vi "SCMP - Data Acquisition - v6.vi"(0 "Max FPS limit":dbl=10.0 format="%.1g", 1 "LCVR Voltages":dbl[][](array[numeric]), 2 "Mod/Seq":bool, 5 "Cycles":i32=1 min=1 max=30 step=1, 7 "Save to FITS?":bool=TRUE, 9 "Headers In":T12[](array[typedef])=[{"Wavelength (nm)"=530.15, "Exposure (s)"=0.05, "Tuning Delay (ms)"=1000.0, "Beam Type (-1/1)"=1.0, "Tuning Voltages"=[1.111, 2.222, 3.333, 4.444], "Observer"="observer", "Light Shapping Diffuser"=enum."In Beam", "Comment"="", "Data Type"=9, "Mod Cycles"=0, "SCD Calibration Optics"=enum."1 - Polarizer @0, I+Q", "SCD Emission Line Filter"=enum."1-557.6nm", "Cookbook"="", "COMP-S Calibration Wheel"=enum."Dark", "COMP-S Andover Filter Wheel"=enum."530.3nm/HWB 0.34nm (Fe XIV)", "FOV Rotation (deg)"=66.0, "Objective Lens Position (mm)"=0.0, "Occulter size"=0.0, "Time End"=timestamp(3382374145.421875 s since 1904-01-01), "Acc Exposure (s)"=0.0, "Time Stamp Array"=[], "Camera Serial Number"=[], "Camera Temp"=[], "Camera PI (mm)"=[], "Time Start"=timestamp(3382374145.421875 s since 1904-01-01), "Peripherals"={"ILX controler"=FALSE, "Zone temperatures"=FALSE, "Andor"=FALSE, "Andor 2"=FALSE, "PI Stages"=FALSE, "AISAS mechanisms"=FALSE, "AISAS Mech.lvclass"=refnum, "Zone temp ref"=variant, "FWs"=FALSE}, "FITS paths"=[], "Cameras"=enum."Andor", "load preset cbk"=FALSE, "periodic check count"=0, "COMP-S Calibration Wheel 2"=enum."Dark", "Calib"=enum."Dark", "Abso Aperture"=40.0, "Nominal Aperture"=196.0}] {"Nominal Aperture" format="%.1f"; "Abso Aperture" format="%.1f"; "Camera PI (mm)" format="%_3g"; "Acc Exposure (s)" format="%^.3g"; "Occulter size" format="%.2f"; "Objective Lens Position (mm)" min=70.0 max=152.0 format="%.2f"; "FOV Rotation (deg)" format="%.1f"; "Data Type" items=["LIVE", "DARK", "FLAT", "CALI", "OBSE", "ABSO", "AURE", "TARG", "OBJE", "HOLE", "OREX", "THRO", "CHIP"]; "Exposure (s)" format="%^.3g"; "Wavelength (nm)" format="%_6g"}, 11 "error in":errorcluster, 12 "Andor Neo":T13[](array[typedef]) {"Exposure (s)" format="%^.3g"; "Time at Synch" format="%<%H:%M:%S>T"; "Interframe Time" format="%#_3g"; "Frame Readout Time" format="%_3g"; "Row Readout Time" format="%_3g"}) -> (3 "FITS Path Out":path, 6 "Image":u32[][](array[numeric]), 8 "Image 2":u32[][](array[numeric]), 10 "Headers Out":T2[](array[typedef]) {"Nominal Aperture" format="%.1f"; "Abso Aperture" format="%.1f"; "Camera PI (mm)" format="%_3g"; "Acc Exposure (s)" format="%^.3g"; "Occulter size" format="%.2f"; "Objective Lens Position (mm)" min=70.0 max=152.0 format="%.2f"; "FOV Rotation (deg)" format="%.1f"; "Exposure (s)" format="%^.3g"; "Wavelength (nm)" format="%_6g"}, 13 "FITS Path Out 2":path, 15 "error out":errorcluster)   [LabVIEW 2014]
doc: "The LL Sequence VI acquires a sequence of images and displays them in an array of image controls using the low-level acquisition VIs. A sequence is appropriate for applications that process multiple images. You can configure a sequence to acquire every frame or to skip a variable number of frames between each image.\n\nTop Level Code Overview\n1) Initialize Camera (Global Shutter, High Well, Low Noise, exposure time, etc.)\n2) Create a buffer set equal in size to the # of trigger pulses (e.g. 100) which is the same as the # of expected images \n3) Start the camera acquisition THEN start the DAQmx task (use merge error cluster to gurantee this)"
uses:
  Controls/run cbk timeout.ctl
  Controls/Globals.vi
  <vilib>/Waveform/WDTOps.llb/WDT Waveform Duration DBL.vi
  <vilib>/DAQmx/write.llb/DAQmx Write (Analog 1D Wfm NChan NSamp).vi
  <vilib>/DAQmx/create/channels.llb/DAQmx Create Channel (AO-Voltage-Basic).vi
  <vilib>/DAQmx/configure/timing.llb/DAQmx Timing (Use Waveform).vi
  Controls/SCD - Calibration Optics Filter Wheel.ctl
  AISAS/Controls/Diffuser.ctl
  Controls/SCD - FITS Cluster.ctl
  Camera/Andor Neo Info.ctl
  Controls/SCD - EDT - Emission Line Filter Wheel.ctl
  Controls/CoMP-S Controls/Polarization Optics Filter Wheel.ctl
  Controls/CoMP-S Controls/Emission Line Filter Wheel.ctl
  AISAS/Controls/focus.ctl
  Controls/beaning.ctl
  AISAS/Mech/AISAS Mech.lvclass
  Controls/peripherals.ctl
  Controls/Cameras select.ctl
  Controls/FITS Data type.ctl
panel:
  out "error Andor queue":errorcluster
  out "error cam dequeue & queue RAM 2":errorcluster
  out "error dequeue RAM 2":errorcluster
  out "seq cycles":i32=1
  out "error proc queue":errorcluster
  out "mod cycles *4":i32=1
  out "error RAM queue":errorcluster
  in  "count 2":i32
  in  "Tab Control":T1(tab)
  out "FPS":dbl=10.0 format="%.1g"
  out "Camera T Image":u32[][](graph)
  out "# Images in queue":i32
  out "Image Acq (s)":dbl(slide)=4151.832132564842
  out "Image Processing":i32(slide) scale=-1.0..11.0
  in  "user break":bool
  out "Camera R Image":u32[][](graph)
  out "Camera T Image Zoom":u32[][](graph)
  out "# Images to acquire":i32
  out "Image Acq Started":bool
  in  "image pointers":u64[](array[numeric])
  in  "imageNo":i32 caption="Image No"
  in  "count":i32
  out "# Wavelengths":i32=1
  out "Exposure (s)":dbl=0.09 format="%_3p"
  out "# elements in cam":i32
  out "Image Cam":u32[][](graph)
  out "# buffer":i32
  in  "image pointers 2":u64[](array[numeric])
  in  "imageNo 2":i32 caption="Image No 2"
  out "# Images in queue 2":i32
  out "# buffer 2":i32
  out "Image transfering":u32(slide) scale=-1.0..88.0
  out "Acquisition Estimate (s)":dbl format="%0.2f"
  out "Image Acq":i32(slide) scale=-1.0..88.0
  out "Image Acq 2":i32(slide) scale=0.0..220.0
  out "Image 2 Procesing":i32(slide) scale=-1.0..11.0
  out "Image transfering 2":u32(slide) scale=0.0..40.0
  out "# elements in cam 2":i32
  out "Actual Wavelength (nm)":dbl format="%.2g"
  out "Time Start":timestamp=timestamp(3382374145.421875 s since 1904-01-01) format="%<%H:%M:%S%3u\n%x>T"
  out "Time stamp arr":timestamp[](array[timestamp]) format="%<%H:%M:%S%3u>T"
  out "COMP Waveforms":waveform(dbl)[](graph)
  out "SCD Waveforms":waveform(dbl)[](graph)
  out "Time stamp arr 2":timestamp[](array[timestamp]) format="%<%H:%M:%S%3u>T"
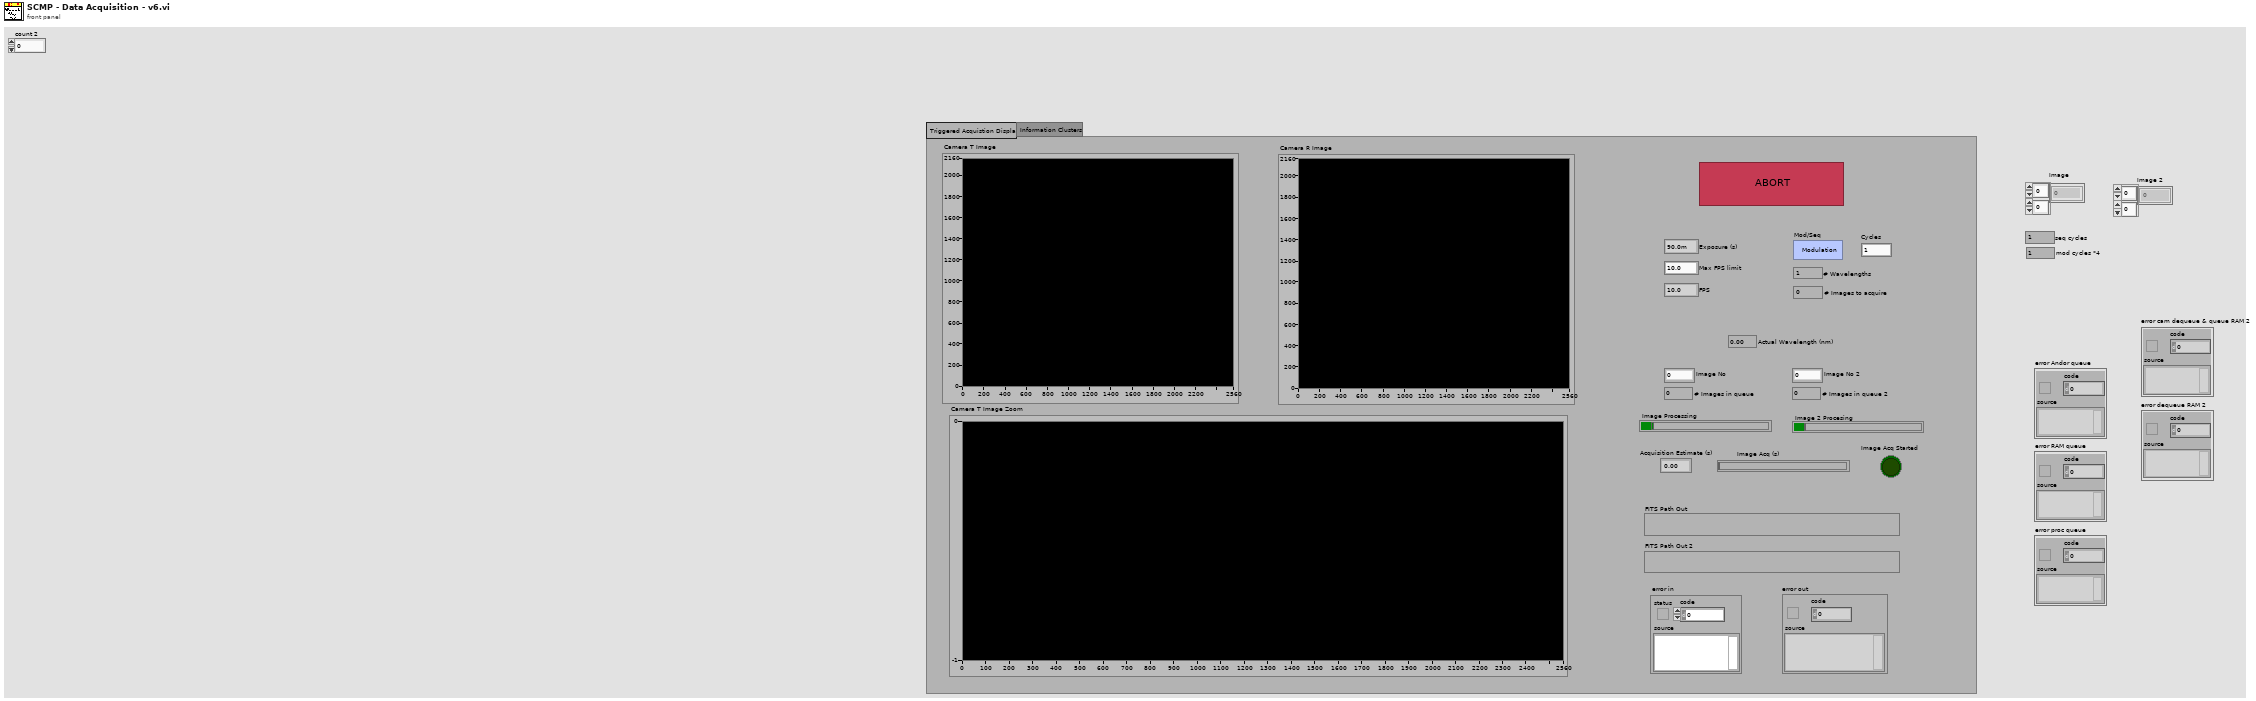
[diagram p1: front panel]
types:
  T1 = enum32{"Triggered Acquistion Display", "Information Clusters"}
  T2 = typedef "SCD - FITS Cluster.ctl" = cluster{"Wavelength (nm)":dbl, "Exposure (s)":dbl, "Tuning Delay (ms)":dbl, "Beam Type (-1/1)":dbl, "Tuning Voltages":dbl[], "Observer":string, "Light Shapping Diffuser":T3, "Comment":string, "Data Type":T4, "Mod Cycles":u16, "SCD Calibration Optics":T5, "SCD Emission Line Filter":T6, "Cookbook":string, "COMP-S Calibration Wheel":T7, "COMP-S Andover Filter Wheel":T8, "FOV Rotation (deg)":dbl, "Objective Lens Position (mm)":T9, "Occulter size":dbl, "Time End":timestamp, "Acc Exposure (s)":dbl, "Time Stamp Array":timestamp[], "Camera Serial Number":string[], "Camera Temp":dbl[], "Camera PI (mm)":dbl[], "Time Start":timestamp, "Peripherals":T10, "FITS paths":path[], "Cameras":T11, "load preset cbk":bool, "periodic check count":i32, "COMP-S Calibration Wheel 2":T7, "Calib":enum16{"Dark", "Flat"}, "Abso Aperture":dbl, "Nominal Aperture":dbl, "Pointer IP":string}
  T3 = typedef "Diffuser.ctl" = enum16{"Out of Beam", "In Beam"}
  T4 = typedef "FITS Data type.ctl" = enum16{"LIVE", "DARK", "FLAT", "CALI", "OBSE", "ABSO", "AURE", "TARG", "OBJE", "HOLE", "OREX", "THRO", "CHIP"}
  T5 = typedef "SCD - Calibration Optics Filter Wheel.ctl" = enum16{"1 - Polarizer @0, I+Q", "2 - Polarizer @90, I-Q", "3 - Polarizer @45, I+U", "4 - Polarizer @135, I-U", "5 - Polarizer @0, Retarder @45, I+V", "6 - Polarizer @0, Retarder @135, I-V", "7 - Dark", "8 - Clear", "9 - N/A"}
  T6 = typedef "SCD - EDT - Emission Line Filter Wheel.ctl" = enum16{"1-557.6nm", "2-587.6nm", "3-589.6nm", "4-630.2nm", "5-656.4nm", "6-849.8nm", "7-854.2nm", "8-866.2nm", "9-1083.0nm"}
  T7 = typedef "Polarization Optics Filter Wheel.ctl" = enum16{"Dark", "Clear", "Exchange Lens", "Polarizer @0, I+Q", "Polarizer @90, I-Q", "Polarizer @45, I+U", "Polarizer @135, I-U", "Polarizer @0, Retarder @45, I+V", "Polarizer @0, Retarder @135, I-V"}
  T8 = typedef "Emission Line Filter Wheel.ctl" = enum16{"530.3nm/HWB 0.34nm (Fe XIV)", "587.6nm/HBW 0.44nm (He I D3)", "637.5nm/HBW 0.53nm (Fe X)", "656.3nm/HBW 0.57nm (H-Alpha)", "789.2nm/HBW 0.85nm (Fe XI)", "854.2nm/HBW 1.01nm (Ca I)", "1074.7nm/HBW 2.34nm (Fe XIII)", "1079.8nm/HBW 1.64nm (Fe XIII)", "1083.0nm/HBW 1.66nm (He I)"}
  T9 = typedef "focus.ctl" = dbl
  T10 = typedef "peripherals.ctl" = cluster{"ILX controler":bool, "Zone temperatures":bool, "Andor":bool, "Andor 2":bool, "PI Stages":bool, "AISAS mechanisms":bool, "AISAS Mech.lvclass":refnum<class "AISAS Mech.lvclass">, "Zone temp ref":variant, "FWs":bool}
  T11 = typedef "Cameras select.ctl" = enum16{"Andor", "GDR"}
  T12 = typedef "SCD - FITS Cluster.ctl" = cluster{"Wavelength (nm)":dbl, "Exposure (s)":dbl, "Tuning Delay (ms)":dbl, "Beam Type (-1/1)":dbl, "Tuning Voltages":dbl[], "Observer":string, "Light Shapping Diffuser":T3, "Comment":string, "Data Type":u16, "Mod Cycles":u16, "SCD Calibration Optics":T5, "SCD Emission Line Filter":T6, "Cookbook":string, "COMP-S Calibration Wheel":T7, "COMP-S Andover Filter Wheel":T8, "FOV Rotation (deg)":dbl, "Objective Lens Position (mm)":T9, "Occulter size":dbl, "Time End":timestamp, "Acc Exposure (s)":dbl, "Time Stamp Array":timestamp[], "Camera Serial Number":string[], "Camera Temp":dbl[], "Camera PI (mm)":dbl[], "Time Start":timestamp, "Peripherals":T10, "FITS paths":path[], "Cameras":T11, "load preset cbk":bool, "periodic check count":i32, "COMP-S Calibration Wheel 2":T7, "Calib":enum16{"Dark", "Flat"}, "Abso Aperture":dbl, "Nominal Aperture":dbl}
  T13 = typedef "Andor Neo Info.ctl" = cluster{"Handle":i32, "Pixel Encoding":string, "AOI Width":i32, "AOI Height":i32, "AOI Stride":i32, "Row Readout Time":dbl, "Frame Readout Time":dbl, "Interframe Time":dbl, "Semaphore":T14, "SerialNumber":string, "Camera Model":string, "Controller ID":string, "Firmware Version":string, "Shutter":string, "BDiv":u8, "Time at Synch":timestamp, "Idx":i32, "PreAmp":string, "Binning":T15, "PixelReadoutRate":string, "Exposure (s)":dbl, "Image Bytes":i64, "Image Pixels":i64, "SpuriousNoiseFilter":bool, "Overlap":bool, "CycleMode":string}
  T14 = typedef "Semaphore RefNum" = refnum<k1>
  T15 = typedef "beaning.ctl" = enum16{"1x1", "2x2", "3x3", "4x4", "8x8"}
  T16 = typedef "run cbk timeout.ctl" = i32
  T17 = enum8{"Enabled", "Disabled", "Disabled and Grayed Out"}
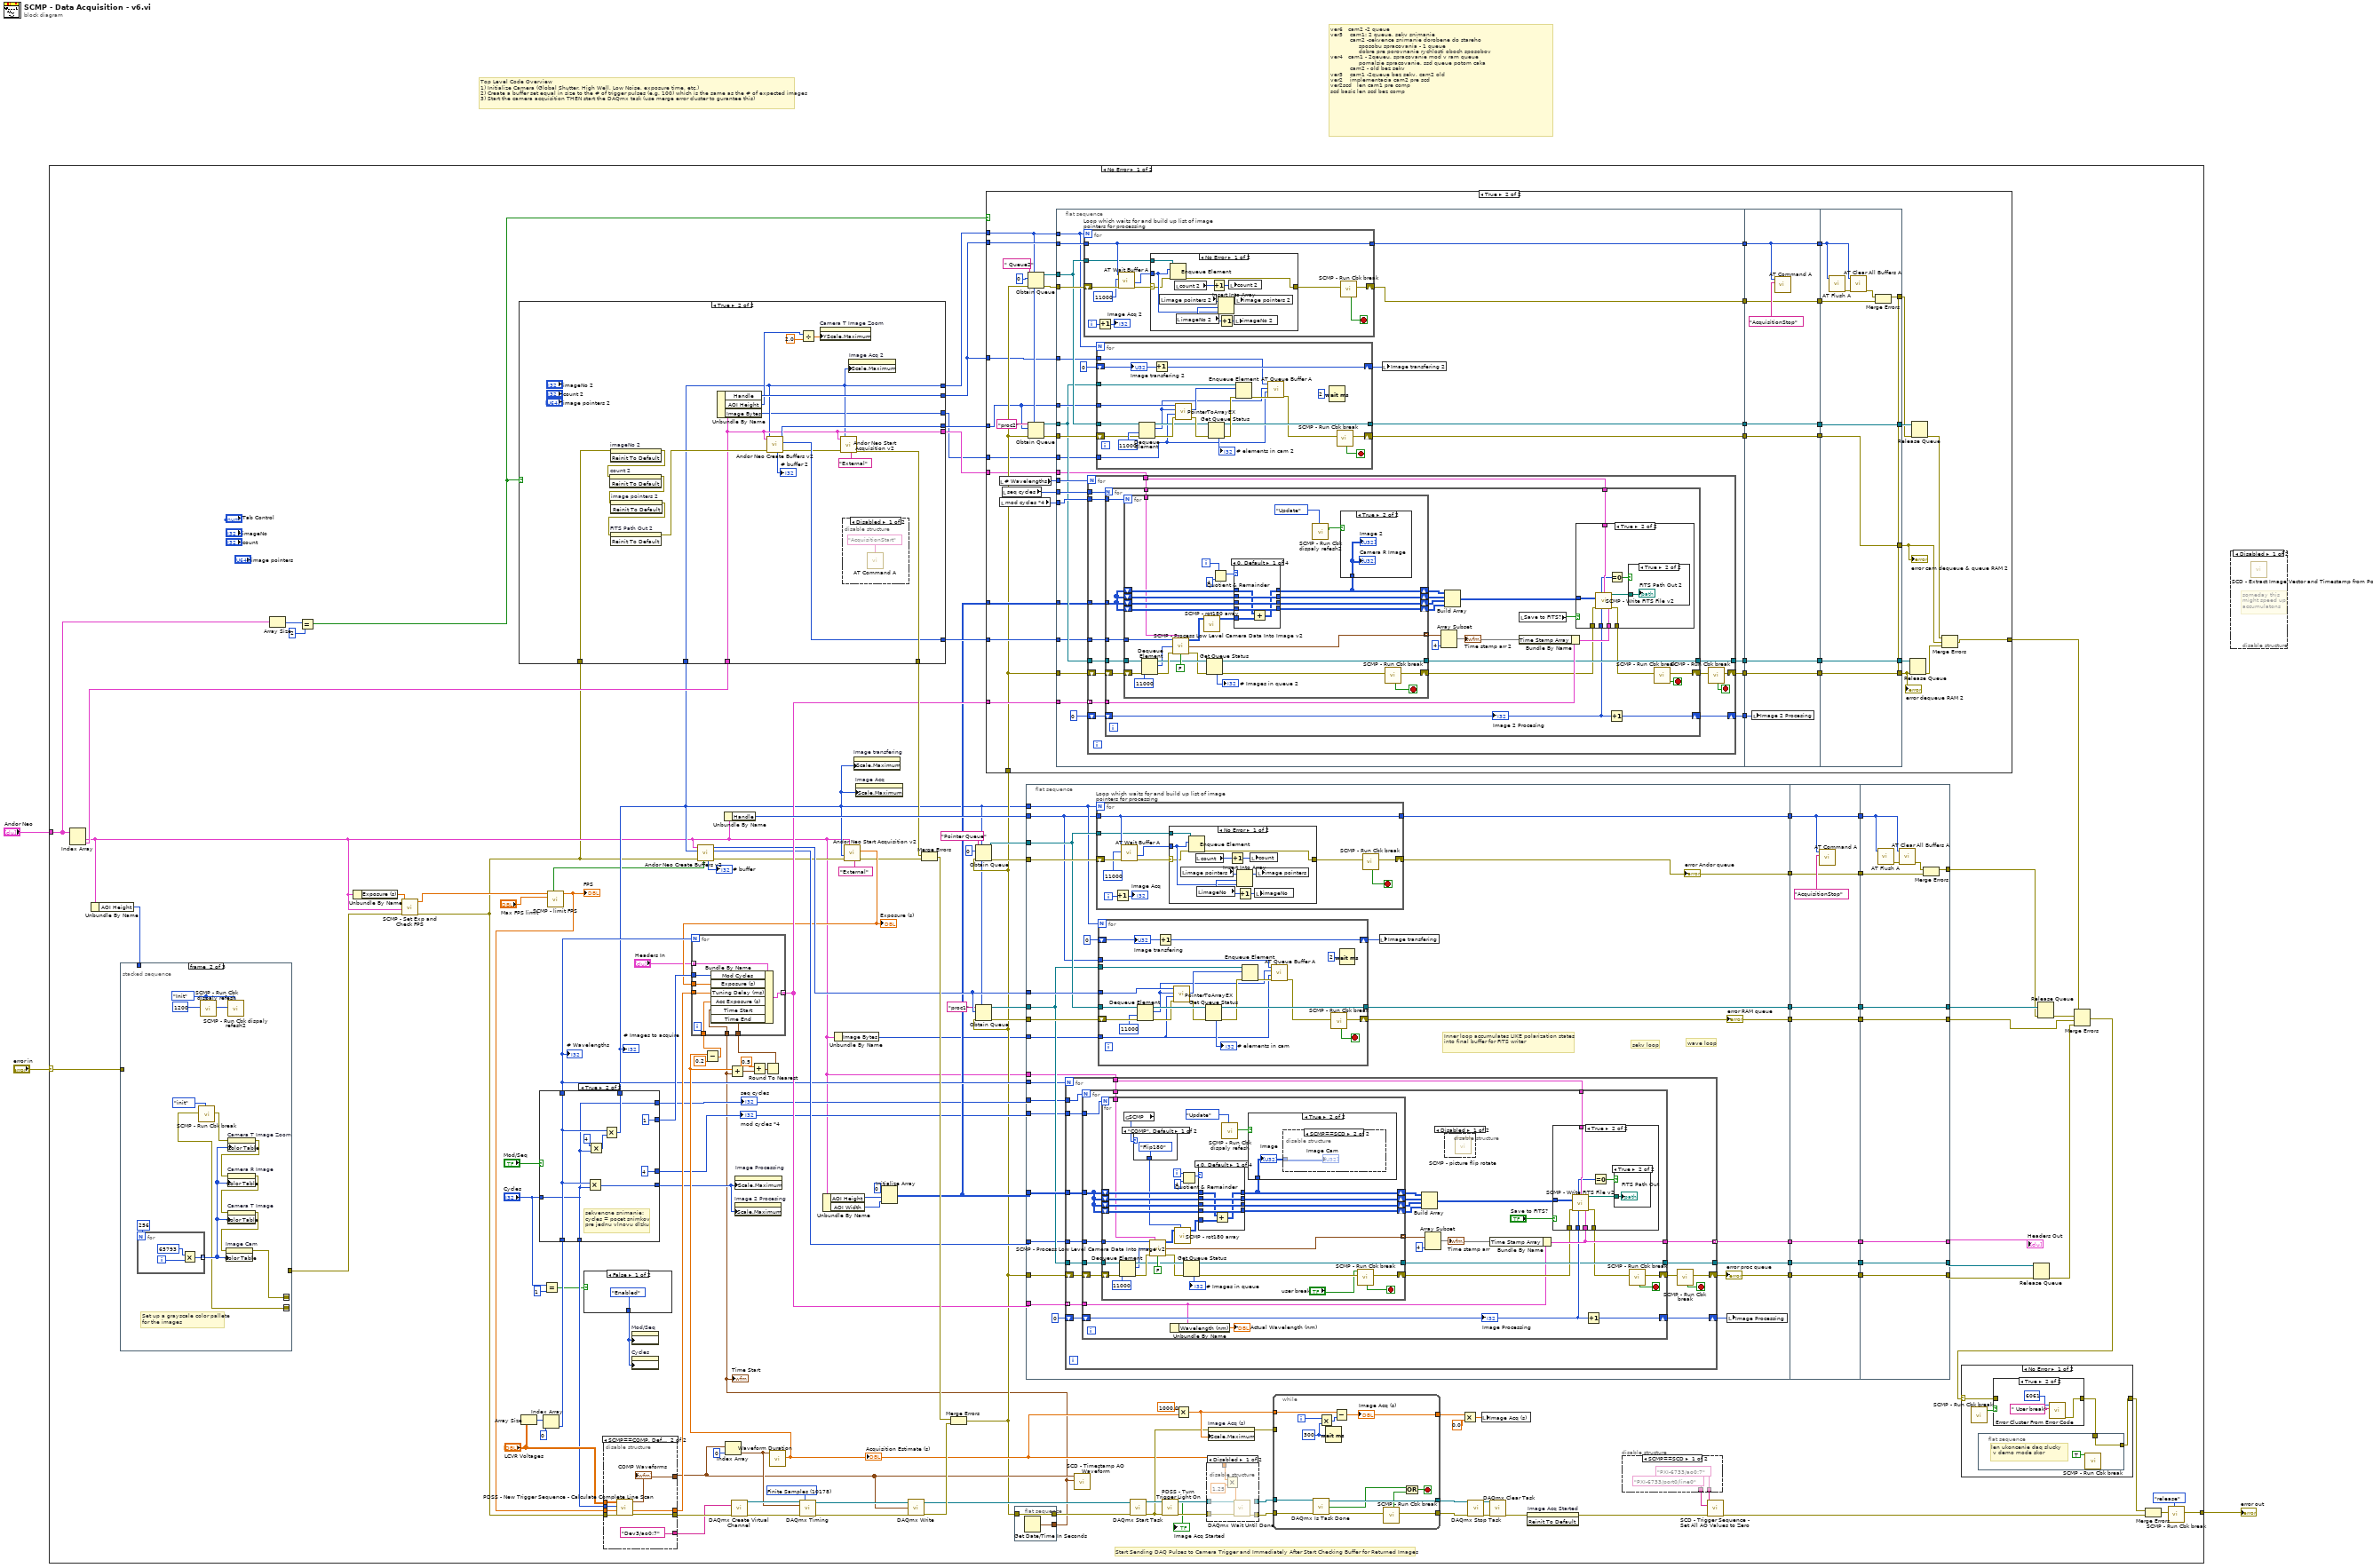
[diagram p0: block diagram]
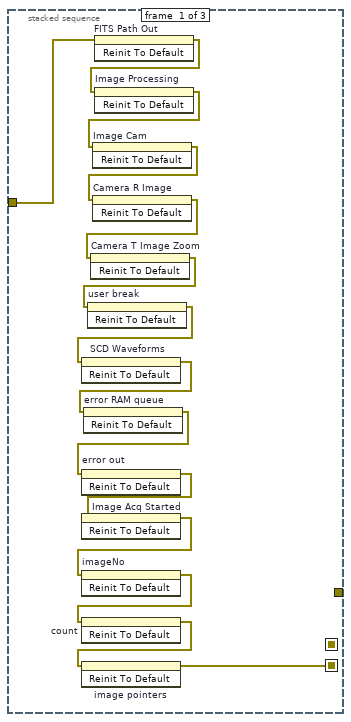
[diagram p3: hidden frame]
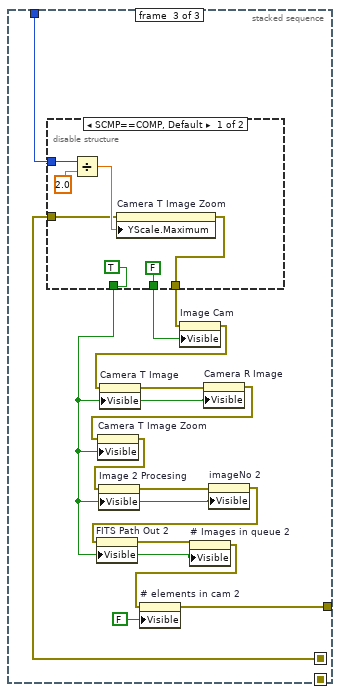
[diagram p4: hidden frame]
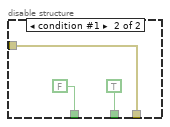
[diagram p5: hidden frame]
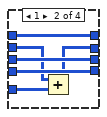
[diagram p8: hidden frame]
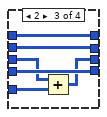
[diagram p9: hidden frame]
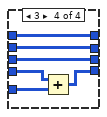
[diagram p10: hidden frame]
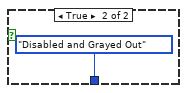
[diagram p16: hidden frame]
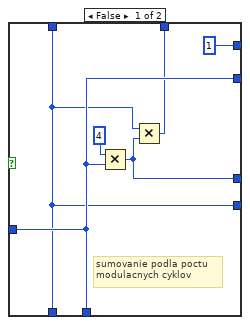
[diagram p20: hidden frame]
diagram:
  # "ver6   cam2 -2 queue\nver5    cam1: 2 queue, sekv snimanie\n           cam2 -sekvence snimanie dorobene do stareho \n                sposobu spracovania - 1 queue \n                dobre pre porovnanie rychlosti oboch sposobov\nver4   cam1 - 2qeueu, spracovanie mod v ram queue\n                pomalsie spracovanie, ssd queue potom caka\n           cam2 - old bez sekv\nver3    cam1 -2queue bez sekv, cam2 old\nver2    implementacia cam2 pre scd\nver2scd   len cam1 pre comp\nscd basic len scd bez comp"
  # "Top Level Code Overview\n1) Initialize Camera (Global Shutter, High Well, Low Noise, exposure time, etc.)\n2) Create a buffer set equal in size to the # of trigger pulses (e.g. 100) which is the same as the # of expected images \n3) Start the camera acquisition THEN start the DAQmx task (use merge error cluster to gurantee this)"
  n1 = case shown="No Error" "error in" {
    selector: "error in" -> [w96 w723]
    tunnel: [w5 w723] -> w3
    tunnel: "Andor Neo" -> [w13 _]
    frame No Error {
      w136 = 10178 items=["Finite Samples"=10178, "Continuous Samples"=10123] ("sample mode")
      # "Start Sending DAQ Pulses to Camera Trigger and Immediately After Start Checking Buffer for Returned Images"
      n2 = Index Array(array=w13) -> (element #1=w11:T13, element #2=w28:T13)  [unwired: 2 in]
      n3 = Unbundle By Name(w11) -> ("AOI Height"=w8:i32)
      n4 = stacked-sequence {
        seq-local: [w139 _ _] -> [_ w152 _]
        seq-local: [_ w156 _] -> [_ _ w166]
        tunnel: w96 -> [w138 _ _]
        tunnel: w8 -> [_ _ w179]
        tunnel: [_ _ w165] -> w7
        frame #0 {
          n5 = invoke on="FITS Path Out" class="Path" method="Reinit To Default"(error in=w138) -> (error out=w137:errorcluster)  [unwired: 2 in, 2 out]
          n6 = invoke on="Image Processing" class="Slide (strict)" method="Reinit To Default"(error in=w137) -> (error out=w148:errorcluster)  [unwired: 2 in, 2 out]
          n7 = invoke on="Image Cam" class="IntGraph (strict)" method="Reinit To Default"(error in=w148) -> (error out=w147:errorcluster)  [unwired: 2 in, 2 out]
          n8 = invoke on="Camera R Image" class="IntGraph (strict)" method="Reinit To Default"(error in=w147) -> (error out=w146:errorcluster)  [unwired: 2 in, 2 out]
          n9 = invoke on="Camera T Image Zoom" class="IntGraph (strict)" method="Reinit To Default"(error in=w146) -> (error out=w149:errorcluster)  [unwired: 2 in, 2 out]
          n10 = invoke on="user break" class="Bool (strict)" method="Reinit To Default"(error in=w149) -> (error out=w150:errorcluster)  [unwired: 2 in, 2 out]
          n11 = invoke on="SCD Waveforms" class="WFGraph (strict)" method="Reinit To Default"(error in=w150) -> (error out=w144:errorcluster)  [unwired: 2 in, 2 out]
          n12 = invoke on="error RAM queue" class="Clust (strict)" method="Reinit To Default"(error in=w144) -> (error out=w145:errorcluster)  [unwired: 2 in, 2 out]
          n13 = invoke on="error out" class="Clust (strict)" method="Reinit To Default"(error in=w145) -> (error out=w140:errorcluster)  [unwired: 2 in, 2 out]
          n14 = invoke on="Image Acq Started" class="Bool (strict)" method="Reinit To Default"(error in=w140) -> (error out=w143:errorcluster)  [unwired: 2 in, 2 out]
          n15 = invoke on="imageNo" class="DigNum (strict)" method="Reinit To Default"(error in=w143) -> (error out=w141:errorcluster)  [unwired: 2 in, 2 out]
          n16 = invoke on="count" class="DigNum (strict)" method="Reinit To Default"(error in=w141) -> (error out=w142:errorcluster)  [unwired: 2 in, 2 out]
          n17 = invoke on="image pointers" class="Arr (strict)" method="Reinit To Default"(error in=w142) -> (error out=w139:errorcluster)  [unwired: 2 in, 2 out]
        }
        frame #1 {
          w153 = enum16{"Init", "Update"}."Init" ("Function")
          w154 = u32 1200 ("Refresh Time")
          # "Set up a grayscale color pallete for the images"
          n18 = for {
            N: 256 -> [_]
            tunnel: [w163] -> w160 mode=indexing
            i -> [w164]
            n19 = Multiply(x=65793, y=w164) -> (x*y=w163:i32)
          }
          n20 = call "SCMP - Run Cbk break.vi"("use/init (use)"=enum16{"use", "init"}."init", "error in (no error)"=w152) -> ("error out"=w151:errorcluster)  [unwired: 7 in, 2 out]
          n21 = call "SCMP - Run Cbk dispaly refesh.vi"("mode"=w153, "Refresh Time {ms}"=w154) -> ()  [unwired: 8 in, 2 out]
          n22 = call "SCMP - Run Cbk dispaly refesh2.vi"("Function"=w153, "Refresh Time {ms}"=w154) -> ()  [unwired: 9 in, 1 out]
          n23 = property on="Camera T Image Zoom" class="IntGraph (strict)"(error in=w151, "Color Table"=w160) -> (error out=w159:errorcluster)  [unwired: 1 in, 1 out]
          n24 = property on="Camera R Image" class="IntGraph (strict)"(error in=w159, "Color Table"=w160) -> (error out=w158:errorcluster)  [unwired: 1 in, 1 out]
          n25 = property on="Camera T Image" class="IntGraph (strict)"(error in=w158, "Color Table"=w160) -> (error out=w157:errorcluster)  [unwired: 1 in, 1 out]
          n26 = property on="Image Cam" class="IntGraph (strict)"(error in=w157, "Color Table"=w160) -> (error out=w156:errorcluster)  [unwired: 1 in, 1 out]
        }
        frame #2 {
          n27 = disable-structure shown="SCMP==COMP, Default" {
            disable-tunnel: w166 -> [w184 w187]
            disable-tunnel: w179 -> [w183 _]
            disable-tunnel: [FALSE ("Visible") TRUE ("Visible")] -> w178
            disable-tunnel: [w181 w187] -> w177
            disable-tunnel: [TRUE ("Visible") FALSE ("Visible")] -> w167
            frame condition #0 (active) {
              n28 = Divide(x=w183, y=2.0) -> (x/y=w186:dbl)
              n29 = property on="Camera T Image Zoom" class="IntGraph (strict)"(error in=w184, "YScale.Maximum"=w186) -> (error out=w181:errorcluster)  [unwired: 1 in, 1 out]
            }
            frame condition #1 {
            }
          }
          n30 = property on="Image Cam" class="IntGraph (strict)"(error in=w177, "Visible"=w178) -> (error out=w175:errorcluster)  [unwired: 1 in, 1 out]
          n31 = property on="Camera T Image" class="IntGraph (strict)"(error in=w175, "Visible"=w167) -> (error out=w174:errorcluster)  [unwired: 1 in, 1 out]
          n32 = property on="Camera R Image" class="IntGraph (strict)"(error in=w174, "Visible"=w167) -> (error out=w173:errorcluster)  [unwired: 1 in, 1 out]
          n33 = property on="Camera T Image Zoom" class="IntGraph (strict)"(error in=w173, "Visible"=w167) -> (error out=w172:errorcluster)  [unwired: 1 in, 1 out]
          n34 = property on="Image 2 Procesing" class="Slide (strict)"(error in=w172, "Visible"=w167) -> (error out=w171:errorcluster)  [unwired: 1 in, 1 out]
          n35 = property on="imageNo 2" class="DigNum (strict)"(error in=w171, "Visible"=w167) -> (error out=w170:errorcluster)  [unwired: 1 in, 1 out]
          n36 = property on="FITS Path Out 2" class="Path"(error in=w170, "Visible"=w167) -> (error out=w169:errorcluster)  [unwired: 1 in, 1 out]
          n37 = property on="# Images in queue 2" class="DigNum (strict)"(error in=w169, "Visible"=w167) -> (error out=w168:errorcluster)  [unwired: 1 in, 1 out]
          n38 = property on="# elements in cam 2" class="DigNum (strict)"(error in=w168, "Visible"=FALSE) -> (error out=w165:errorcluster)  [unwired: 1 in, 1 out]
        }
      }
      n39 = Array Size(array=w13) -> (size(s)=w27:i32)
      n40 = Equal?(x=w27, y=2) -> (x = y?=w25:bool)
      n41 = Unbundle By Name(w11) -> ("Exposure (s)"=w12:dbl)
      n42 = call "SCMP - Set Exp and Check FPS.vi"("Andor"=w11, "error in (no error)"=w7, "Exposure [s]"=w12) -> ("error out"=w9:errorcluster, "FPS"=w10:dbl)  [unwired: 7 in]
      n43 = Array Size(array="LCVR Voltages") -> (size(s)=w122:i32[])
      n44 = Index Array(array=w122, index=0) -> (element=w64:i32)
      n45 = case shown="True" "Mod/Seq" {
        tunnel: [w467 4] -> w45
        tunnel: [w465 w474] -> w23
        tunnel: [w463 w471] -> w47
        tunnel: w64 -> [w463 w471]
        tunnel: [w466 1 ("Cycles")] -> w66
        tunnel: [w466 w469] -> w65
        tunnel: "Cycles" -> [w466 w469]
        tunnel: [w463 w470] -> w43
        tunnel: [1 ("value") w469] -> w44
        frame False {
          # "sumovanie podla poctu\nmodulacnych cyklov"
          n46 = Multiply(x=4 ("value"), y=w466) -> (x*y=w467:i32)
          n47 = Multiply(x=w463, y=w467) -> (x*y=w465:i32)
        }
        frame True {
          # "sekvencne snimanie:\ncycles = pocet snimkov\npre jednu vlnovu dlzku"
          n48 = Multiply(x=w471, y=w469) -> (x*y=w470:i32)
          n49 = Multiply(x=4 ("value"), y=w469) -> (x*y=w475:i32)
          n50 = Multiply(x=w471, y=w475) -> (x*y=w474:i32)
        }
      }
      "# Wavelengths" <- w47
      "# Images to acquire" <- w23
      "mod cycles *4" <- w45
      "seq cycles" <- w44
      n51 = case shown="True" w25 {
        tunnel: [_ w440] -> w85
        tunnel: [_ w439] -> w22
        tunnel: [_ w438] -> w82
        tunnel: [_ w425] -> w81
        tunnel: w9 -> [_ w437]
        tunnel: [_ w436] -> w42
        tunnel: [_ w426] -> w29
        tunnel: w28 -> [_ w426]
        tunnel: w23 -> [_ w425]
        tunnel: [_ w424] -> w21
        frame False {
        }
        frame True {
          n52 = invoke on="imageNo 2" class="DigNum (strict)" method="Reinit To Default"(error in=w437) -> (error out=w435:errorcluster)  [unwired: 2 in, 2 out]
          n53 = invoke on="count 2" class="DigNum (strict)" method="Reinit To Default"(error in=w435) -> (error out=w434:errorcluster)  [unwired: 2 in, 2 out]
          n54 = invoke on="image pointers 2" class="Arr (strict)" method="Reinit To Default"(error in=w434) -> (error out=w433:errorcluster)  [unwired: 2 in, 2 out]
          n55 = invoke on="FITS Path Out 2" class="Path" method="Reinit To Default"(error in=w433) -> (error out=w432:errorcluster)  [unwired: 2 in, 2 out]
          n56 = Unbundle By Name(w426) -> ("Handle"=w439:i32, "AOI Height"=w429:i32, "Image Bytes"=w424:i64)
          n57 = call "Andor Neo Create Buffers v2.vi"("error in"=w432, "Number of Images"=w425, "Camera Info"=w426) -> ("error out"=w428:errorcluster, "PixelData"=w438:i64[], "ByteData"=w436:u8[], "# of Andor buffers"=→"# buffer 2":i32)  [unwired: 4 in, 1 out]
          n58 = Divide(x=w429, y=2.0) -> (x/y=w431:dbl)
          n59 = property on="Camera T Image Zoom" class="IntGraph (strict)"("YScale.Maximum"=w431) -> ()  [unwired: 2 in, 2 out]
          n60 = call "Andor Neo Start Acquisition v2.vi"("TriggerMode"="External" ("TriggerMode 2"), "error in"=w428, "Frames"=w425, "Andor in"=w426) -> ("error out"=w440:errorcluster)  [unwired: 5 in, 2 out]
          n61 = disable-structure shown="Disabled" {
            frame Disabled {
              n62 = call <userlib>:"AT Command A.vi"("Feature"="AcquisitionStart" ("Command")) -> ()  [unwired: 9 in, 2 out]
            }
            frame Enabled {
            }
          }
          n63 = property on="Image Acq 2" class="Slide (strict)"("Scale.Maximum"=w425) -> ()  [unwired: 2 in, 2 out]
        }
      }
      n64 = Equal?(x="Cycles", y=1) -> (x = y?=w53:bool)
      n65 = case shown="False" w53 {
        tunnel: [T17."Enabled" ("Disabled") T17."Disabled and Grayed Out" ("Disabled")] -> w17
        frame False {
        }
        frame True {
        }
      }
      n66 = property on="Mod/Seq" class="Bool (strict)"("DisabledEnum"=w17) -> ()  [unwired: 2 in, 2 out]
      n67 = property on="Cycles" class="DigNum (strict)"("DisabledEnum"=w17) -> ()  [unwired: 2 in, 2 out]
      n68 = call "Andor Neo Create Buffers v2.vi"("error in"=w9, "Number of Images"=w23, "Camera Info"=w11) -> ("error out"=w38:errorcluster, "PixelData"=w48:i64[], "ByteData"=w52:u8[], "# of Andor buffers"=→"# buffer":i32, "circural buffer?"=w15:bool)  [unwired: 4 in]
      n69 = call "SCMP - limit FPS.vi"("circural buffer?"=w15, "Max FPS limit in"="Max FPS limit", "FPS in"=w10) -> ("FPS out"=w14:dbl)  [unwired: 8 in]
      "FPS" <- w14
      n70 = disable-structure shown="SCMP==COMP, Default" {
        disable-tunnel: [w497 w502] -> w129
        disable-tunnel: "LCVR Voltages" -> [w496 w505]
        disable-tunnel: [w491 w500] -> w103
        disable-tunnel: w14 -> [w495 w498]
        disable-tunnel: w9 -> [w494 w503]
        disable-tunnel: [w493 w501] -> w104
        disable-tunnel: w65 -> [w492 w504]
        disable-tunnel: [tag "PXI-6733/ao0:7" ("physical channels") tag "Dev3/ao0:7" ("physical channels")] -> w90
        frame condition #0 {
          n71 = call "SCD - Trigger Sequence Generation - Complete Recipe.vi"("error in"=w494, "FPS"=w495, "Modulation Cycles\nAt Each Wavelength"=w492, "LCVR Voltages"=w496) -> ("error out"=w497:errorcluster, "LCVR Relaxtion Time"=w493:dbl, "SCD Waveforms (Graph)"=w491:waveform(dbl)[])  [unwired: 5 in]
          "SCD Waveforms" <- w491
        }
        frame condition #1 (active) {
          n72 = call "PDSS - New Trigger Sequence - Calculate Complete Line Scan.vi"("error in"=w503, "FPS"=w498, "Modulation Cycles\nAt Each Wavelength"=w504, "LCVR Voltages"=w505) -> ("error out"=w502:errorcluster, "LCVR Relaxtion Time"=w501:dbl, "AO Graph"=w500:waveform(dbl)[])  [unwired: 5 in]
          "COMP Waveforms" <- w500
        }
      }
      n73 = Unbundle By Name(w11) -> ("Handle"=w88:i32)
      n74 = Index Array(array=w103, index=0) -> (element=w126:waveform(dbl))
      n75 = call-poly <vilib>:"DAQmx Create Virtual Channel.vi"("physical channels"=w90, "error in"=w129) -> ("task out"=w134:refnum<k21>, "error out"=w135:errorcluster)  [unwired: 12 in]
      n76 = property on="Image 2 Procesing" class="Slide (strict)"("Scale.Maximum"=w43) -> ()  [unwired: 2 in, 2 out]
      n77 = property on="Image Processing" class="Slide (strict)"("Scale.Maximum"=w43) -> ()  [unwired: 2 in, 2 out]
      n78 = call-poly <vilib>:"Waveform Duration.vi"("waveform in"=w126) -> ("duration"=w61:dbl)  [unwired: 8 in, 2 out]
      "Acquisition Estimate (s)" <- w61
      n79 = Subtract(x=w61, y=0.2) -> (x-y=w97:dbl)
      n80 = Add(x=w61, y=w34) -> (x+y=w33:timestamp)
      n81 = Add(x=0.5, y=w33) -> (x+y=w32:timestamp)
      n82 = Round To Nearest(number=w32) -> (nearest integer value=w41:timestamp)
      n83 = call-poly <vilib>:"DAQmx Timing.vi"("task/channels in"=w134, "sample mode"=w136, "waveform"=w126, "error in"=w135) -> ("task out"=w127:refnum<k21>, "error out"=w128:errorcluster)  [unwired: 10 in]
      n84 = Unbundle By Name(w11) -> ("AOI Height"=w50:i32, "AOI Width"=w49:i32)
      n85 = Unbundle By Name(w11) -> ("Image Bytes"=w24:i64)
      n86 = call "Andor Neo Start Acquisition v2.vi"("TriggerMode"="External" ("TriggerMode 2"), "error in"=w38, "Frames"=w23, "Andor in"=w11) -> ("error out"=w37:errorcluster, "Exposure Get"=w39:dbl)  [unwired: 5 in, 1 out]
      "Exposure (s)" <- w39
      n87 = for {
        N: w47 -> [_]
        tunnel: [w517] -> w84 mode=indexing
        tunnel: w39 -> [w516]
        tunnel: "Headers In" -> [w515] mode=indexing
        tunnel: w104 -> [w514]
        tunnel: w66 -> [w513]
        tunnel: w97 -> [w512]
        tunnel: w41 -> [w511]
        tunnel: w34 -> [w510]
        n88 = Bundle By Name(cluster=w515, "Mod Cycles"=w513, "Exposure (s)"=w516, "Tuning Delay (ms)"=w514, "Acc Exposure (s)"=w512, "Time Start"=w510, "Time End"=w511) -> (w517:T12)
      }
      n89 = property on="Image transfering" class="Slide (strict)"("Scale.Maximum"=w23) -> ()  [unwired: 2 in, 2 out]
      n90 = property on="Image Acq" class="Slide (strict)"("Scale.Maximum"=w23) -> ()  [unwired: 2 in, 2 out]
      n91 = Initialize Array(u32 0, w50, w49) -> (w46:u32[][])
      n92 = call-poly <vilib>:"DAQmx Write.vi"("task/channels in"=w127, "data"=w103, "error in"=w128) -> ("task out"=w87:refnum<k21>, "error out"=w116:errorcluster)  [unwired: 10 in, 1 out]
      n93 = Merge Errors(w85, w37) -> (w86:errorcluster)
      n94 = Merge Errors(w86, w116) -> (w35:errorcluster)
      n95 = Obtain Queue(max queue size (-1, unlimited)=w23, name (unnamed)="Pointer Queue", element data type=u64 0 ("Output buffer"), error in (no error)=w35) -> (queue out=w110:refnum<queue>, error out=w111:errorcluster)  [unwired: 1 in, 1 out]
      n96 = Obtain Queue(max queue size (-1, unlimited)=w23, name (unnamed)="proc1", element data type=w52, error in (no error)=w35) -> (queue out=w51:refnum<queue>, error out=w75:errorcluster)  [unwired: 1 in, 1 out]
      n97 = case shown="True" w25 {
        tunnel: w84 -> [_ w216]
        tunnel: [_ w215] -> w83
        tunnel: w22 -> [_ w214]
        tunnel: w82 -> [_ w213]
        tunnel: w81 -> [_ w212]
        tunnel: w46 -> [_ w211]
        tunnel: w42 -> [_ w191]
        tunnel: w35 -> [_ w210]
        tunnel: w29 -> [_ w209]
        tunnel: w22 -> [_ w192]
        tunnel: w21 -> [_ w190]
        frame False {
        }
        frame True {
          n98 = local read "# Wavelengths"() -> (w204:i32)
          n99 = local read "mod cycles *4"() -> (w202:i32)
          n100 = local read "seq cycles"() -> (w201:i32)
          n101 = Obtain Queue(max queue size (-1, unlimited)=w212, name (unnamed)=" Queue2", element data type=u64 0 ("Output buffer"), error in (no error)=w210) -> (queue out=w206:refnum<queue>, error out=w205:errorcluster)  [unwired: 1 in, 1 out]
          n102 = Obtain Queue(max queue size (-1, unlimited)=w212, name (unnamed)="proc2", element data type=w191, error in (no error)=w210) -> (queue out=w199:refnum<queue>, error out=w200:errorcluster)  [unwired: 1 in, 1 out]
          n103 = flat-sequence {
            tunnel: w205 -> [w256]
            tunnel: w214 -> [w255]
            tunnel: [w254] -> w229
            tunnel: [w253] -> w228
            tunnel: w209 -> [w235]
            tunnel: w213 -> [w240]
            tunnel: w206 -> [w252]
            tunnel: [w238] -> w227
            tunnel: w202 -> [w244]
            tunnel: [w237] -> w226
            tunnel: w212 -> [w249]
            tunnel: w216 -> [w243]
            tunnel: w204 -> [w246]
            tunnel: w211 -> [w239]
            tunnel: w201 -> [w245]
            tunnel: w200 -> [w248]
            tunnel: w191 -> [w247]
            tunnel: w199 -> [w241]
            tunnel: [w236] -> w225
            tunnel: [w234] -> w224
            tunnel: [w233] -> w223
            tunnel: w210 -> [w232]
            tunnel: w192 -> [w231]
            tunnel: w190 -> [w230]
            tunnel: w229 -> [w410]
            tunnel: w228 -> [w409]
            tunnel: w227 -> [w412]
            tunnel: w226 -> [w411]
            tunnel: [w410] -> w222
            tunnel: [w412] -> w221
            tunnel: [w411] -> w220
            tunnel: [w409] -> w219
            tunnel: w225 -> [w408]
            tunnel: [w407] -> w218
            tunnel: w224 -> [w407]
            tunnel: [w406] -> w217
            tunnel: w223 -> [w406]
            tunnel: [w422] -> _
            tunnel: [w421] -> w195
            tunnel: w222 -> [w419]
            tunnel: w221 -> [w417]
            tunnel: w220 -> [w422]
            tunnel: w219 -> [w420]
            tunnel: [w417] -> w203
            tunnel: w218 -> [w416]
            tunnel: [w416] -> w194
            tunnel: [w415] -> w198
            tunnel: w217 -> [w415]
            frame #0 {
              n104 = for "Loop which waits for and build up list of image pointers for processing" {
                N: w249 -> [_]
                tunnel: w255 -> [w392]
                tunnel: [w392] -> w254
                tunnel: w252 -> [w390]
                shift-right: [w385] -> w253
                shift-left: w256 -> [w394]
                i -> [w388]
                stop <- w384 stop-if-true
                n105 = Increment(x=w388) -> (x+1=→"Image Acq 2":i32)
                n106 = call <userlib>:"AT Wait Buffer A.vi"("error in (no error)"=w394, "Timeout"=T16 11000 ("timeout for deque loop"), "Handle"=w392) -> ("error out"=w391:errorcluster, "Output buffer"=w393:u64)  [unwired: 5 in, 2 out]
                n107 = case shown="No Error" w391 {
                  selector: w391 -> [w396 w405]
                  tunnel: w393 -> [w398 _]
                  tunnel: [w395 w405] -> w386
                  tunnel: w390 -> [w397 _]
                  frame No Error {
                    n108 = local read "image pointers 2"() -> (w402:u64[])
                    n109 = Enqueue Element(queue=w397, element=w398, error in (no error)=w396) -> (error out=w395:errorcluster)  [unwired: 1 in, 2 out]
                    n110 = local read "count 2"() -> (w404:i32)
                    n111 = local read "imageNo 2"() -> (w399:i32)
                    n112 = Increment(x=w404) -> (x+1=w403:i32)
                    n113 = Insert Into Array(array=w402, index=w399, new element=w398) -> (w401:u64[])
                    n114 = Increment(x=w399) -> (x+1=w400:i32)
                    n115 = local write "count 2"(w403) -> ()
                    n116 = local write "imageNo 2"(w400) -> ()
                    n117 = local write "image pointers 2"(w401) -> ()
                  }
                  frame Error {
                  }
                }
                n118 = call "SCMP - Run Cbk break.vi"("error in (no error)"=w386) -> ("error out"=w385:errorcluster, "stop ack"=w384:bool)  [unwired: 8 in, 1 out]
              }
              n119 = for {
                N: w246 -> [_]
                tunnel: w243 -> [w270] mode=indexing
                tunnel: w235 -> [w263]
                shift-right: [w258] -> w237
                shift-left: w232 -> [w269]
                tunnel: w241 -> [w268]
                tunnel: [w267] -> w238
                shift-right: [w266] -> w236
                shift-left: 0 ("Image SSD Saving 2") -> [w265]
                tunnel: w239 -> [w264]
                tunnel: w240 -> [w262]
                tunnel: w245 -> [w261]
                tunnel: w244 -> [w260]
                stop <- w257 stop-if-true
                n120 = for {
                  N: w261 -> [_]
                  tunnel: w263 -> [w293]
                  shift-right: [w272] -> w259
                  shift-left: w269 -> [w290]
                  shift-right: [w292] -> w266
                  shift-left: w265 -> [w275]
                  tunnel: w270 -> [w295]
                  tunnel: w268 -> [w289]
                  tunnel: [w288] -> w267
                  tunnel: w264 -> [w291]
                  tunnel: w263 -> [w283]
                  tunnel: w262 -> [w277]
                  tunnel: w260 -> [w276]
                  stop <- w271 stop-if-true
                  n121 = for {
                    N: w276 -> [_]
                    shift-right: [w309] -> w282
                    shift-left: w291 -> [w324]
                    shift-right: [w320] -> w281
                    shift-left: w291 -> [w323]
                    shift-right: [w319] -> w280
                    shift-left: w291 -> [w322]
                    shift-right: [w318] -> w279
                    shift-left: w291 -> [w321]
                    shift-right: [w297] -> w287
                    shift-left: w290 -> [w317]
                    tunnel: w289 -> [w304]
                    tunnel: [w311] -> w288
                    tunnel: [w310] -> w285 mode=indexing
                    tunnel: w283 -> [w308]
                    tunnel: w277 -> [w306]
                    i -> [w303]
                    stop <- w296 stop-if-true
                    n122 = Dequeue Element(queue=w304, timeout in ms (-1)=T16 11000 ("timeout for deque loop"), error in (no error)=w317) -> (queue out=w313:refnum<queue>, element=w307:u8[], error out=w314:errorcluster)  [unwired: 1 out]
                    n123 = call "SCMP - Process Low Level Camera Data Into Image v2.vi"("PixelData (U16)"=w306, "Andor Cluster"=w308, "Input buffer"=w307, "error in (no error)"=w314, "Demo pic \n(Andor/SCMP)"=FALSE ("scmp demo pic")) -> ("Image (I32)"=w300:u32[][], "Timestamp"=w310:timestamp, "error out"=w312:errorcluster)  [unwired: 8 in]
                    n124 = call "SCMP - rot180 array.vi"("A in"=w300) -> ("A out"=w301:u32[][])  [unwired: 10 in]
                    n125 = Get Queue Status(queue=w313, error in (no error)=w312) -> (queue out=w311:refnum<queue>, error out=w298:errorcluster, # elements in queue=→"# Images in queue 2":i32)  [unwired: 1 in, 5 out]
                    n126 = Quotient & Remainder(x=w303, y=4) -> (x-y*floor(x/y)=w325:i32)  [unwired: 1 out]
                    n127 = case shown="0, Default" w325 {
                      tunnel: w321 -> [w331 w338 w344 w347]
                      tunnel: w322 -> [w332 w339 w341 w350]
                      tunnel: w323 -> [w333 w335 w345 w351]
                      tunnel: w324 -> [w329 w336 w342 w348]
                      tunnel: [w328 w336 w342 w348] -> w309
                      tunnel: [w333 w334 w345 w351] -> w320
                      tunnel: [w332 w339 w340 w350] -> w319
                      tunnel: [w331 w338 w344 w346] -> w318
                      tunnel: w301 -> [w330 w337 w343 w349]
                      frame 0, Default {
                        n128 = Add(x=w329, y=w330) -> (x+y=w328:u32[][])
                      }
                      frame 1 {
                        n129 = Add(x=w335, y=w337) -> (x+y=w334:u32[][])
                      }
                      frame 2 {
                        n130 = Add(x=w341, y=w343) -> (x+y=w340:u32[][])
                      }
                      frame 3 {
                        n131 = Add(x=w347, y=w349) -> (x+y=w346:u32[][])
                      }
                    }
                    n132 = call "SCMP - Run Cbk dispaly refesh2.vi"("Function"=enum16{"Init", "Update", "Stop"}."Update") -> ("Display Refresh"=w302:bool)  [unwired: 10 in]
                    n133 = case shown="True" w302 {
                      tunnel: w309 -> [_ w327]
                      frame False {
                      }
                      frame True {
                        "Image 2" <- w327
                        "Camera R Image" <- w327
                      }
                    }
                    n134 = call "SCMP - Run Cbk break.vi"("error in (no error)"=w298) -> ("error out"=w297:errorcluster, "stop ack"=w296:bool)  [unwired: 8 in, 1 out]
                  }
                  n135 = Array Subset(array=w285, length=4) -> (w284:timestamp[])  [unwired: 1 in]
                  "Time stamp arr 2" <- w284
                  n136 = Build Array(w282, w281, w280, w279) -> (w278:u32[][][])
                  n137 = local read "Save to FITS?"() -> (w274:bool)
                  n138 = Bundle By Name(cluster=w295, "Time Stamp Array"=w284) -> (w294:T12)
                  n139 = case shown="True" w274 {
                    tunnel: w294 -> [_ w360]
                    tunnel: w293 -> [_ w359]
                    tunnel: w275 -> [_ w358]
                    tunnel: [w352 w355] -> w273
                    tunnel: w287 -> [w352 w354]
                    tunnel: w278 -> [_ w353]
                    frame False {
                    }
                    frame True {
                      n140 = call "SCMP - Write FITS File v2.vi"("FITS Header"=w360, "Andor"=w359, "Data"=w353, "error in"=w354, "Image #"=w358) -> ("FITS Path Out"=w356:path, "error out"=w355:errorcluster)  [unwired: 8 in, 1 out]
                      n141 = Equal To 0?(x=w358) -> (x = 0?=w357:bool)
                      n142 = case shown="True" w357 {
                        tunnel: w356 -> [_ w361]
                        frame False {
                        }
                        frame True {
                          "FITS Path Out 2" <- w361
                        }
                      }
                    }
                  }
                  n143 = Increment(x=w275) -> (x+1=w292:i32)
                  n144 = call "SCMP - Run Cbk break.vi"("error in (no error)"=w273) -> ("error out"=w272:errorcluster, "stop ack"=w271:bool)  [unwired: 8 in, 1 out]
                  "Image 2 Procesing" <- w275
                }
                n145 = call "SCMP - Run Cbk break.vi"("error in (no error)"=w259) -> ("error out"=w258:errorcluster, "stop ack"=w257:bool)  [unwired: 8 in, 1 out]
              }
              n146 = for {
                N: w249 -> [_]
                tunnel: w252 -> [w377]
                shift-right: [w375] -> w250
                shift-left: u32 0 ("Image transfering") -> [w376]
                shift-right: [w363] -> w234
                shift-left: w248 -> [w374]
                tunnel: w247 -> [w373]
                tunnel: w241 -> [w372]
                tunnel: [w370] -> w233
                tunnel: w231 -> [w367]
                tunnel: w230 -> [w366]
                stop <- w362 stop-if-true
                n147 = Dequeue Element(queue=w377, timeout in ms (-1)=T16 11000 ("timeout for deque loop"), error in (no error)=w374) -> (queue out=w371:refnum<queue>, element=w368:u64, error out=w380:errorcluster)  [unwired: 1 out]
                n148 = Increment(x=w376) -> (x+1=w375:u32)
                n149 = call <userlib>:"PointerToArrayEX.vi"("Array in"=w373, "Pointer In"=w368, "Pointer Size"=w366, "error in (no error)"=w380) -> ("Array out"=w378:u8[], "error out"=w379:errorcluster)  [unwired: 4 in]
                n150 = Get Queue Status(queue=w371, error in (no error)=w379) -> (queue out=w370:refnum<queue>, error out=w383:errorcluster, # elements in queue=→"# elements in cam 2":i32)  [unwired: 1 in, 5 out]
                n151 = Enqueue Element(queue=w372, element=w378, error in (no error)=w383) -> (error out=w369:errorcluster)  [unwired: 1 in, 2 out]
                n152 = call <userlib>:"AT Queue Buffer A.vi"("error in (no error)"=w369, "PtrSize"=w366, "Ptr"=w368, "Handle"=w367) -> ("error out"=w364:errorcluster)  [unwired: 6 in, 1 out]
                n153 = Wait (ms)(milliseconds to wait=u32 2) -> ()  [unwired: 1 out]
                n154 = call "SCMP - Run Cbk break.vi"("error in (no error)"=w364) -> ("error out"=w363:errorcluster, "stop ack"=w362:bool)  [unwired: 8 in, 1 out]
                "Image transfering 2" <- w376
              }
              n155 = local write "Image transfering 2"(w250) -> ()
            }
            frame #1 {
              n156 = local write "Image 2 Procesing"(w408) -> ()
              n157 = call <userlib>:"AT Command A.vi"("Feature"="AcquisitionStop" ("Command"), "Handle"=w410) -> ()  [unwired: 8 in, 2 out]
            }
            frame #2 {
              n158 = call <userlib>:"AT Flush A.vi"("Handle"=w419) -> ("error out"=w414:errorcluster)  [unwired: 9 in, 1 out]
              n159 = call <userlib>:"AT Clear All Buffers A.vi"("error in (no error)"=w414, "Handle"=w419) -> ("error out"=w418:errorcluster)  [unwired: 8 in, 1 out]
              n160 = Merge Errors(w418, w420) -> (w421:errorcluster)
            }
          }
          n161 = Release Queue(queue=w203, error in (no error)=w195) -> (error out=w197:errorcluster)  [unwired: 1 in, 2 out]
          n162 = Release Queue(queue=w198, error in (no error)=w195) -> (error out=w196:errorcluster)  [unwired: 1 in, 2 out]
          n163 = Merge Errors(w196, w194, w197) -> (w215:errorcluster)
          "error dequeue RAM 2" <- w195
          "error cam dequeue & queue RAM 2" <- w194
        }
      }
      n164 = flat-sequence {
        tunnel: [w519] -> w114
        tunnel: w35 -> [w519]
        tunnel: [w518] -> w34
        frame #0 {
          n165 = Get Date/Time In Seconds() -> (seconds since 1Jan1904=w518:timestamp)
        }
      }
      n166 = flat-sequence {
        tunnel: w111 -> [w546]
        tunnel: w23 -> [w529]
        tunnel: w88 -> [w524]
        tunnel: [w545] -> w118
        tunnel: [w520] -> w117
        tunnel: w84 -> [w542]
        tunnel: [w541] -> w113
        tunnel: w52 -> [w544]
        tunnel: w110 -> [w539]
        tunnel: [w543] -> w108
        tunnel: [w521] -> w101
        tunnel: w75 -> [w540]
        tunnel: [w522] -> w74
        tunnel: [w538] -> w72
        tunnel: w46 -> [w533]
        tunnel: w51 -> [w532]
        tunnel: w11 -> [w531]
        tunnel: w48 -> [w530]
        tunnel: w47 -> [w528]
        tunnel: w44 -> [w527]
        tunnel: w45 -> [w526]
        tunnel: w35 -> [w525]
        tunnel: w24 -> [w523]
        tunnel: w118 -> [w708]
        tunnel: w117 -> [w707]
        tunnel: w113 -> [w711]
        tunnel: w108 -> [w710]
        tunnel: w101 -> [w709]
        tunnel: [w708] -> w95
        tunnel: [w711] -> w94
        tunnel: [w710] -> w93
        tunnel: [w709] -> w92
        tunnel: [w707] -> w91
        tunnel: w74 -> [w706]
        tunnel: [w706] -> w73
        tunnel: w72 -> [w705]
        tunnel: [w705] -> w71
        tunnel: [w720] -> w89
        tunnel: [w721] -> w107
        tunnel: [w722] -> w105
        tunnel: [w719] -> w106
        tunnel: w95 -> [w717]
        tunnel: w94 -> [w722]
        tunnel: w93 -> [w721]
        tunnel: w92 -> [w720]
        tunnel: w91 -> [w718]
        tunnel: w73 -> [w715]
        tunnel: [w715] -> w68
        tunnel: w71 -> [w714]
        tunnel: [w714] -> w70
        frame #0 {
          # "wave loop"
          # "sekv loop"
          # "Inner loop accumulates LIKE polarization states into final buffer for FITS writer"
          n167 = for {
            N: w528 -> [_]
            tunnel: w542 -> [w561] mode=indexing
            tunnel: [w560] -> w541 mode=indexing
            tunnel: w531 -> [w553]
            shift-right: [w548] -> w522
            shift-left: w525 -> [w559]
            tunnel: w532 -> [w558]
            tunnel: [w557] -> w538
            shift-right: [w556] -> w535
            shift-left: 0 -> [w555]
            tunnel: w533 -> [w554]
            tunnel: w530 -> [w552]
            tunnel: w527 -> [w551]
            tunnel: w526 -> [w550]
            stop <- w547 stop-if-true
            n168 = for {
              N: w551 -> [_]
              tunnel: w553 -> [w586]
              shift-right: [w563] -> w549
              shift-left: w559 -> [w581]
              shift-right: [w584] -> w556
              shift-left: w555 -> [w583]
              tunnel: w561 -> [w566]
              tunnel: [w587] -> w560
              tunnel: w558 -> [w580]
              tunnel: [w579] -> w557
              tunnel: w554 -> [w582]
              tunnel: w553 -> [w574]
              tunnel: w552 -> [w568]
              tunnel: w550 -> [w567]
              stop <- w562 stop-if-true
              n169 = for {
                N: w567 -> [_]
                shift-right: [w601] -> w573
                shift-left: w582 -> [w618]
                shift-right: [w614] -> w572
                shift-left: w582 -> [w617]
                shift-right: [w613] -> w571
                shift-left: w582 -> [w616]
                shift-right: [w612] -> w570
                shift-left: w582 -> [w615]
                shift-right: [w590] -> w578
                shift-left: w581 -> [w611]
                tunnel: w580 -> [w610]
                tunnel: [w604] -> w579
                tunnel: [w602] -> w576 mode=indexing
                tunnel: w574 -> [w600]
                tunnel: w568 -> [w598]
                i -> [w619]
                stop <- w588 stop-if-true
                n170 = Dequeue Element(queue=w610, timeout in ms (-1)=T16 11000 ("timeout for deque loop"), error in (no error)=w611) -> (queue out=w606:refnum<queue>, element=w599:u8[], error out=w607:errorcluster)  [unwired: 1 out]
                n171 = global read "Globals.vi" "SCMP"() -> (w594:enum16{"COMP", "SCD"})
                n172 = case shown="\"COMP\", Default" w594 {
                  tunnel: [enum16{"noop", "Rot180", "Flip180"}."Flip180" ("op") enum16{"noop", "Rot180", "Flip180"}."Rot180" ("op")] -> w593
                  frame "COMP", Default {
                  }
                  frame "SCD" {
                  }
                }
                n173 = call "SCMP - Process Low Level Camera Data Into Image v2.vi"("PixelData (U16)"=w598, "Andor Cluster"=w600, "Input buffer"=w599, "error in (no error)"=w607, "Demo pic \n(Andor/SCMP)"=FALSE ("scmp demo pic")) -> ("Image (I32)"=w596:u32[][], "Timestamp"=w602:timestamp, "error out"=w605:errorcluster)  [unwired: 8 in]
                n174 = call "SCMP - rot180 array.vi"("pic op (noop)"=w593, "A in"=w596) -> ("A out"=w595:u32[][])  [unwired: 9 in]
                n175 = Quotient & Remainder(x=w619, y=4) -> (x-y*floor(x/y)=w620:i32)  [unwired: 1 out]
                n176 = Get Queue Status(queue=w606, error in (no error)=w605) -> (queue out=w604:refnum<queue>, error out=w591:errorcluster, # elements in queue=→"# Images in queue":i32)  [unwired: 1 in, 5 out]
                n177 = case shown="0, Default" w620 {
                  tunnel: w615 -> [w630 w637 w643 w646]
                  tunnel: w616 -> [w631 w638 w640 w649]
                  tunnel: w617 -> [w632 w634 w644 w650]
                  tunnel: w618 -> [w628 w635 w641 w647]
                  tunnel: [w627 w635 w641 w647] -> w601
                  tunnel: [w632 w633 w644 w650] -> w614
                  tunnel: [w631 w638 w639 w649] -> w613
                  tunnel: [w630 w637 w643 w645] -> w612
                  tunnel: w595 -> [w629 w636 w642 w648]
                  frame 0, Default {
                    n178 = Add(x=w628, y=w629) -> (x+y=w627:u32[][])
                  }
                  frame 1 {
                    n179 = Add(x=w634, y=w636) -> (x+y=w633:u32[][])
                  }
                  frame 2 {
                    n180 = Add(x=w640, y=w642) -> (x+y=w639:u32[][])
                  }
                  frame 3 {
                    n181 = Add(x=w646, y=w648) -> (x+y=w645:u32[][])
                  }
                }
                n182 = call "SCMP - Run Cbk dispaly refesh.vi"("mode"=enum16{"Init", "Update", "Stop"}."Update" ("Function")) -> ("Display Refresh"=w597:bool)  [unwired: 9 in, 1 out]
                n183 = case shown="True" w597 {
                  tunnel: w601 -> [_ w624]
                  frame False {
                  }
                  frame True {
                    n184 = disable-structure shown="SCMP==SCD" {
                      disable-tunnel: w624 -> [w625 w626]
                      frame condition #0 (active) {
                        "Camera T Image Zoom" <- w625
                        "Camera T Image" <- w625
                      }
                      frame condition #1 {
                        "Image Cam" <- w626
                      }
                    }
                    "Image" <- w624
                  }
                }
                n185 = call "SCMP - Run Cbk break.vi"("error in (no error)"=w591, "user break"="user break") -> ("error out"=w590:errorcluster, "stop ack"=w588:bool)  [unwired: 7 in, 1 out]
              }
              n186 = Unbundle By Name(w566) -> ("Wavelength (nm)"=→"Actual Wavelength (nm)":dbl)
              n187 = Build Array(w573, w572, w571, w570) -> (w569:u32[][][])
              n188 = Array Subset(array=w576, length=4) -> (w575:timestamp[])  [unwired: 1 in]
              "Time stamp arr" <- w575
              n189 = disable-structure shown="Disabled" {
                frame Disabled {
                  n190 = call "SCMP - picture flip rotate.vi"() -> ()  [unwired: 8 in, 4 out]
                }
                frame Enabled {
                }
              }
              n191 = Bundle By Name(cluster=w566, "Time Stamp Array"=w575) -> (w587:T12)
              n192 = case shown="True" "Save to FITS?" {
                tunnel: w587 -> [_ w659]
                tunnel: w586 -> [_ w658]
                tunnel: w583 -> [_ w657]
                tunnel: [w651 w654] -> w564
                tunnel: w578 -> [w651 w653]
                tunnel: w569 -> [_ w652]
                frame False {
                }
                frame True {
                  n193 = call "SCMP - Write FITS File v2.vi"("FITS Header"=w659, "Andor"=w658, "Data"=w652, "error in"=w653, "Image #"=w657) -> ("FITS Path Out"=w655:path, "error out"=w654:errorcluster)  [unwired: 8 in, 1 out]
                  n194 = Equal To 0?(x=w657) -> (x = 0?=w656:bool)
                  n195 = case shown="True" w656 {
                    tunnel: w655 -> [_ w660]
                    frame False {
                    }
                    frame True {
                      "FITS Path Out" <- w660
                    }
                  }
                }
              }
              n196 = Increment(x=w583) -> (x+1=w584:i32)
              n197 = call "SCMP - Run Cbk break.vi"("error in (no error)"=w564) -> ("error out"=w563:errorcluster, "stop ack"=w562:bool)  [unwired: 8 in, 1 out]
              "Image Processing" <- w583
            }
            n198 = call "SCMP - Run Cbk break.vi"("error in (no error)"=w549) -> ("error out"=w548:errorcluster, "stop ack"=w547:bool)  [unwired: 8 in, 1 out]
          }
          "error proc queue" <- w522
          n199 = for "Loop which waits for and build up list of image pointers for processing" {
            N: w529 -> [_]
            tunnel: w524 -> [w691]
            tunnel: [w691] -> w545
            tunnel: w539 -> [w689]
            shift-right: [w684] -> w520
            shift-left: w546 -> [w693]
            i -> [w688]
            stop <- w683 stop-if-true
            n200 = Increment(x=w688) -> (x+1=→"Image Acq":i32)
            n201 = call <userlib>:"AT Wait Buffer A.vi"("error in (no error)"=w693, "Timeout"=T16 11000 ("timeout for deque loop"), "Handle"=w691) -> ("error out"=w690:errorcluster, "Output buffer"=w692:u64)  [unwired: 5 in, 2 out]
            n202 = case shown="No Error" w690 {
              selector: w690 -> [w695 w704]
              tunnel: w692 -> [w697 _]
              tunnel: [w694 w704] -> w685
              tunnel: w689 -> [w696 _]
              frame No Error {
                n203 = local read "image pointers"() -> (w701:u64[])
                n204 = Enqueue Element(queue=w696, element=w697, error in (no error)=w695) -> (error out=w694:errorcluster)  [unwired: 1 in, 2 out]
                n205 = local read "count"() -> (w703:i32)
                n206 = local read "imageNo"() -> (w698:i32)
                n207 = Increment(x=w703) -> (x+1=w702:i32)
                n208 = Insert Into Array(array=w701, index=w698, new element=w697) -> (w700:u64[])
                n209 = Increment(x=w698) -> (x+1=w699:i32)
                n210 = local write "count"(w702) -> ()
                n211 = local write "imageNo"(w699) -> ()
                n212 = local write "image pointers"(w700) -> ()
              }
              frame Error {
              }
            }
            n213 = call "SCMP - Run Cbk break.vi"("error in (no error)"=w685) -> ("error out"=w684:errorcluster, "stop ack"=w683:bool)  [unwired: 8 in, 1 out]
          }
          "error Andor queue" <- w520
          n214 = for {
            N: w529 -> [_]
            tunnel: w544 -> [w681]
            shift-right: [w662] -> w521
            shift-left: w540 -> [w679]
            tunnel: w539 -> [w682]
            tunnel: [w680] -> w543
            tunnel: w532 -> [w677]
            shift-right: [w670] -> w534
            shift-left: u32 0 ("Image transfering") -> [w671]
            tunnel: w524 -> [w666]
            tunnel: w523 -> [w665]
            stop <- w661 stop-if-true
            n215 = Dequeue Element(queue=w682, timeout in ms (-1)=T16 11000 ("timeout for deque loop"), error in (no error)=w679) -> (queue out=w676:refnum<queue>, element=w667:u64, error out=w673:errorcluster)  [unwired: 1 out]
            n216 = Increment(x=w671) -> (x+1=w670:u32)
            n217 = call <userlib>:"PointerToArrayEX.vi"("Array in"=w681, "Pointer In"=w667, "Pointer Size"=w665, "error in (no error)"=w673) -> ("Array out"=w669:u8[], "error out"=w672:errorcluster)  [unwired: 4 in]
            n218 = Get Queue Status(queue=w676, error in (no error)=w672) -> (queue out=w680:refnum<queue>, error out=w678:errorcluster, # elements in queue=→"# elements in cam":i32)  [unwired: 1 in, 5 out]
            n219 = Enqueue Element(queue=w677, element=w669, error in (no error)=w678) -> (error out=w668:errorcluster)  [unwired: 1 in, 2 out]
            n220 = call <userlib>:"AT Queue Buffer A.vi"("error in (no error)"=w668, "PtrSize"=w665, "Ptr"=w667, "Handle"=w666) -> ("error out"=w663:errorcluster)  [unwired: 6 in, 1 out]
            n221 = call "SCMP - Run Cbk break.vi"("error in (no error)"=w663) -> ("error out"=w662:errorcluster, "stop ack"=w661:bool)  [unwired: 8 in, 1 out]
            n222 = Wait (ms)(milliseconds to wait=u32 2) -> ()  [unwired: 1 out]
            "Image transfering" <- w671
          }
          "error RAM queue" <- w521
          n223 = local write "Image transfering"(w534) -> ()
          n224 = local write "Image Processing"(w535) -> ()
        }
        frame #1 {
          n225 = call <userlib>:"AT Command A.vi"("Feature"="AcquisitionStop" ("Command"), "Handle"=w708) -> ()  [unwired: 8 in, 2 out]
        }
        frame #2 {
          n226 = call <userlib>:"AT Flush A.vi"("Handle"=w717) -> ("error out"=w713:errorcluster)  [unwired: 9 in, 1 out]
          n227 = call <userlib>:"AT Clear All Buffers A.vi"("error in (no error)"=w713, "Handle"=w717) -> ("error out"=w716:errorcluster)  [unwired: 8 in, 1 out]
          n228 = Merge Errors(w716, w718) -> (w719:errorcluster)
        }
      }
      n229 = call "SCD - Timestamp AO Waveform.vi"("DAQ To"=w34, "SCD AO Waveforms"=w103) -> ()  [unwired: 8 in, 2 out]
      n230 = call <vilib>:"DAQmx Start Task.vi"("task/channels in"=w87, "error in"=w114) -> ("task out"=w133:refnum<k21>, "error out"=w78:errorcluster)  [unwired: 12 in]
      n231 = call "PDSS - Turn Trigger Light On.vi"("error in (no error)"=w78) -> ("error out"=w125:errorcluster, "Trigger Started"=→"Image Acq Started":bool)  [unwired: 9 in]
      n232 = Multiply(x=1000.0, y=w61) -> (x*y=w79:dbl)
      n233 = disable-structure shown="Disabled" {
        disable-tunnel: w133 -> [w460 w462]
        disable-tunnel: w125 -> [w459 w461]
        disable-tunnel: [w457 w461] -> w63
        disable-tunnel: w61 -> [w455 _]
        disable-tunnel: [_ w462] -> w60
        frame Disabled {
          n234 = Multiply(x=w455, y=1.25 ("x")) -> (x*y=w458:dbl)
          n235 = call <vilib>:"DAQmx Wait Until Done.vi"("task/channels in"=w460, "timeout (sec)"=w458, "error in"=w459) -> ("error out"=w457:errorcluster)  [unwired: 11 in, 1 out]
        }
        frame Enabled {
        }
      }
      n236 = property on="Image Acq (s)" class="Slide (strict)"(error in=w78, "Scale.Maximum"=w79) -> (error out=w77:errorcluster)  [unwired: 1 in, 1 out]
      n237 = while {
        tunnel: w79 -> [w483]
        tunnel: w77 -> [_]
        tunnel: w63 -> [w486]
        tunnel: [w479] -> w62
        tunnel: w60 -> [w485]
        tunnel: [w484] -> w59
        tunnel: [w482] -> w58
        i -> [w488]
        stop <- w481 stop-if-true
        w487 = u32 300 ("milliseconds to wait")
        n238 = call <vilib>:"DAQmx Is Task Done.vi"("task/channels in"=w485, "error in"=w486) -> ("task out"=w484:refnum<k21>, "task done?"=w478:bool, "error out"=w480:errorcluster)  [unwired: 11 in]
        n239 = Multiply(x=w488, y=w487) -> (x*y=w489:u32)
        n240 = Wait (ms)(milliseconds to wait=w487) -> ()  [unwired: 1 out]
        n241 = Subtract(x=w483, y=w489) -> (x-y=w482:dbl)
        "Image Acq (s)" <- w482
        n242 = call "SCMP - Run Cbk break.vi"("error in (no error)"=w480) -> ("error out"=w479:errorcluster, "stop ack"=w477:bool)  [unwired: 8 in, 1 out]
        n243 = Or(x=w478, y=w477) -> (x .or. y?=w481:bool)
      }
      n244 = Multiply(x=w58, y=0.0 ("Image Acq (s)")) -> (x*y=w57:dbl)
      n245 = call <vilib>:"DAQmx Stop Task.vi"("task/channels in"=w59, "error in"=w62) -> ("task out"=w132:refnum<k21>, "error out"=w131:errorcluster)  [unwired: 12 in]
      n246 = local write "Image Acq (s)"(w57) -> ()
      n247 = call <vilib>:"DAQmx Clear Task.vi"("task in"=w132, "error in"=w131) -> ("error out"=w120:errorcluster)  [unwired: 13 in]
      n248 = invoke on="Image Acq Started" class="Bool (strict)" method="Reinit To Default"(error in=w120) -> (error out=w119:errorcluster)  [unwired: 2 in, 2 out]
      n249 = disable-structure shown="SCMP==SCD" {
        disable-tunnel: [tag "PXI-6733/port0/line0" ("lines") tag "Dev3/port0/line0" ("comp lines")] -> w100
        disable-tunnel: [tag "PXI-6733/ao0:7" ("physical channels") tag "Dev3/ao0:7" ("physical channels")] -> w99
        frame condition #0 {
        }
        frame condition #1 (active) {
        }
      }
      n250 = call "SCD - Trigger Sequence - Set All AO Values to Zero.vi"("error in"=w119, "lines"=w100, "physical channels"=w99) -> ("error out"=w115:errorcluster)  [unwired: 8 in]
      n251 = Release Queue(queue=w70, error in (no error)=w68) -> (error out=w69:errorcluster)  [unwired: 1 in, 2 out]
      n252 = Release Queue(queue=w107, error in (no error)=w106) -> (error out=w102:errorcluster)  [unwired: 1 in, 2 out]
      n253 = Merge Errors(w83, w102, w89, w69) -> (w19:errorcluster)
      n254 = case shown="No Error" w19 {
        selector: w19 -> [w447 w454]
        tunnel: [w445 w454] -> w18
        frame No Error {
          n255 = call "SCMP - Run Cbk break.vi"() -> ("stop ack"=w444:bool)  [unwired: 9 in, 2 out]
          n256 = flat-sequence {
            tunnel: w446 -> [w448]
            tunnel: [w448] -> w445
            frame #0 {
              # "len ukoncenie daq slucky\n v demo mode skor"
              n257 = call "SCMP - Run Cbk break.vi"("user break"=TRUE ("break in")) -> ()  [unwired: 8 in, 3 out]
            }
          }
          n258 = case shown="True" w444 {
            tunnel: w447 -> [w450 _]
            tunnel: [w450 w451] -> w446
            frame False {
            }
            frame True {
              n259 = call <vilib>:"Error Cluster From Error Code.vi"("error message (\"\")"=" User break" ("error message (\"\")"), "error code (0)"=6061) -> ("error out"=w451:errorcluster)  [unwired: 7 in]
            }
          }
        }
        frame Error {
        }
      }
      n260 = Merge Errors(w18, w115) -> (w6:errorcluster)
      n261 = call "SCMP - Run Cbk break.vi"("use/init (use)"=enum16{"use", "init", "release"}."release", "error in (no error)"=w6) -> ("error out"=w5:errorcluster)  [unwired: 7 in, 2 out]
      "Headers Out" <- w105
      "Time Start" <- w34
    }
    frame Error {
    }
  }
  "error out" <- w3
  n262 = disable-structure shown="Disabled" {
    frame Disabled {
      # "someday this\nmight speed up\naccumulatons"
      n263 = call "SCD - Extract Image Vector and Timestamp from Pointer.vi"() -> ()  [unwired: 13 in, 3 out]
    }
    frame Enabled {
    }
  }
